vi "PID Relay Out.vi"(0 "Setpoint Reference":dbl=20.0 format="%.2f", 1 "Relay Setpoint":bool, 5 "Relay Amplitude":dbl format="%.2f", 7 "Process Variable":dbl=20.0 format="%.2f", 9 "Noise Disturbance":dbl format="%.2f", 12 "Process Variable Reference":dbl=20.0 format="%.2f") -> (4 "relay output":dbl=50.0 format="%.2f", 6 "Zero Crossing":bool)   [LabVIEW 2017, in "NI_PID_autopid.lvlib"]
doc: "This function relays the setpoint between (setpoint - relay amplitude) and (setpoint + relay amplitude)."
uses:
  <vilib>/addons/control/pid/NI_PID_autopid.lvlib
panel:
  # "Relay Out"
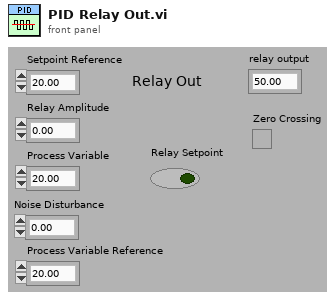
[diagram p1: front panel]
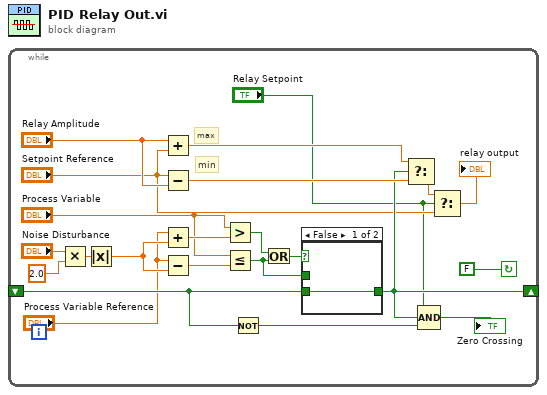
[diagram p0: block diagram]
diagram:
  n1 = while {
    shift-left: _ -> [w8]
    shift-right: [w7] -> _
    stop <- FALSE continue-if-true
    # "min"
    # "max"
    n2 = Multiply(x="Noise Disturbance", y=2.0) -> (x*y=w20:dbl)
    n3 = Absolute Value(x=w20) -> (abs(x)=w16:dbl)
    n4 = Add(x="Relay Amplitude", y="Setpoint Reference") -> (x+y=w12:dbl)
    n5 = Subtract(x="Setpoint Reference", y="Relay Amplitude") -> (x-y=w11:dbl)
    n6 = Add(x="Process Variable Reference", y=w16) -> (x+y=w23:dbl)
    n7 = Subtract(x="Process Variable Reference", y=w16) -> (x-y=w15:dbl)
    n8 = Greater?(x="Process Variable", y=w23) -> (0:w13:bool)
    n9 = Less Or Equal?(x="Process Variable", y=w15) -> (x <= y?=w9:bool)
    n10 = Not(x=w8) -> (.not. x?=w21:bool)
    n11 = Or(x=w13, y=w9) -> (x .or. y?=w10:bool)
    n12 = case shown="False" w10 {
      tunnel: w8 -> [w24 _]
      tunnel: [w24 w25] -> w7
      tunnel: w9 -> [_ w25]
      frame False {
      }
      frame True {
      }
    }
    n13 = Select(t=w12, s=w7, f=w11) -> (s? t:f=w4:dbl)
    n14 = Compound Arithmetic op=AND("Relay Setpoint", w7, w21) -> (→"Zero Crossing":bool)
    n15 = Select(t=w4, s="Relay Setpoint", f="Setpoint Reference") -> (s? t:f=→"relay output":dbl)
  }
